vi "Write applicationElements.vi"(10 "applicationElements":T1, 11 "Model in":refnum<class "Model.lvclass">) -> (3 "Model out":refnum<class "Model.lvclass">)   [LabVIEW 2015, in "Model.lvclass"]
uses:
  Model.lvclass
  ApplicationElements/ApplicationElements.ctl
  ApplicationElements/SystemController/SystemController.lvclass
  ApplicationElements/TestMonitor/TestMonitor.lvclass
  ApplicationElements/StiffnessMonitor/StiffnessMonitor.lvclass
  ApplicationElements/Log/TestDataLog/TestDataLog.lvclass
  ApplicationElements/DistanceGaugeTC/DistanceGaugeTC.lvclass
  ApplicationElements/ForceSensorCalculatorTC/ForceSensorCalculatorTC.lvclass
  ApplicationElements/PressureValveTC/PressureValveTC.lvclass
  ApplicationElements/StiffnessCalculator/StiffnessCalculator.lvclass
  ApplicationElements/PreconditioningMonitor/PreconditioningMonitor.lvclass
  Model.lvclass/Model.ctl
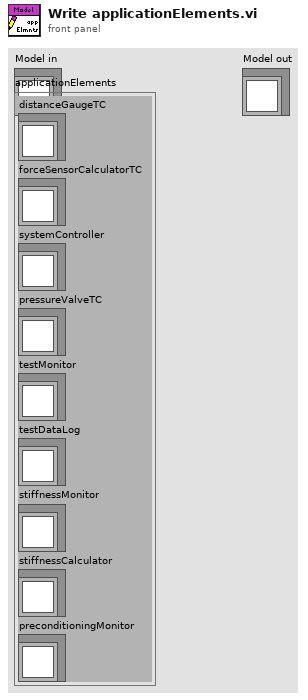
[diagram p1: front panel]
types:
  T1 = typedef "ApplicationElements.ctl" = cluster{"distanceGaugeTC":refnum<class "DistanceGaugeTC.lvclass">, "forceSensorCalculatorTC":refnum<class "ForceSensorCalculatorTC.lvclass">, "systemController":refnum<class "SystemController.lvclass">, "pressureValveTC":refnum<class "PressureValveTC.lvclass">, "testMonitor":refnum<class "TestMonitor.lvclass">, "testDataLog":refnum<class "TestDataLog.lvclass">, "stiffnessMonitor":refnum<class "StiffnessMonitor.lvclass">, "stiffnessCalculator":refnum<class "StiffnessCalculator.lvclass">, "preconditioningMonitor":refnum<class "PreconditioningMonitor.lvclass">}
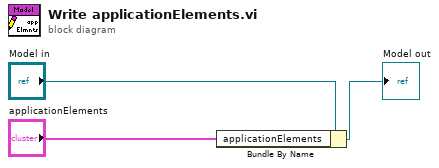
[diagram p0: block diagram]
diagram:
  n1 = Bundle By Name(cluster="Model in", "applicationElements"="applicationElements") -> (→"Model out":refnum<class "Model.lvclass">)
